vi "sub get keyword value.vi"(8 "error in":errorcluster, 10 "keyword":string[](array[string]), 11 "string":string) -> (0 "error out":errorcluster, 2 "matched pairs (exist)":cluster{"keyword":string, "value":string}[](array[cluster]), 3 "matched pairs (all)":cluster{"keyword":string, "value":string}[](array[cluster]), 5 "remain string":string)   [LabVIEW 2018, in "Data Parser.lvclass"]
uses:
  Data Parser.lvclass
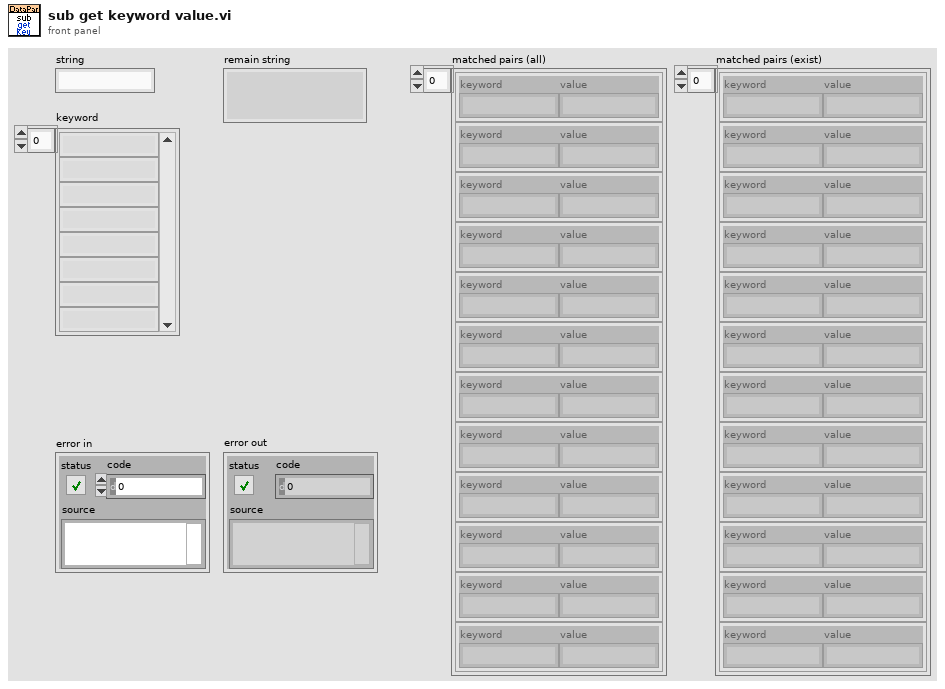
[diagram p1: front panel]
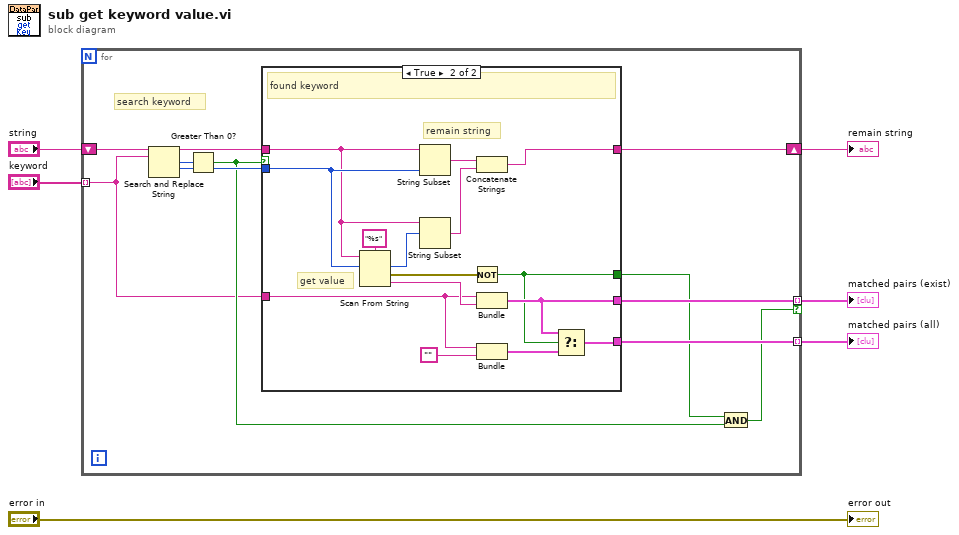
[diagram p0: block diagram]
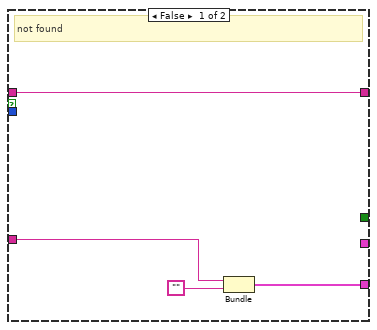
[diagram p2: hidden frame]
diagram:
  n1 = for {
    tunnel: "keyword" -> [w8] mode=indexing
    shift-right: [w14] -> w3
    shift-left: "string" -> [w17]
    tunnel: [w13] -> w6 mode=indexing if=w9
    tunnel: [w12] -> w1 mode=indexing
    # "search keyword"
    n2 = Search and Replace String(input string=w17, search string=w8) -> (result string=w15:string, number of replacements=w11:i32, offset past replacement=w16:i32)  [unwired: 6 in, 1 out]
    n3 = Greater Than 0?(x=w11) -> (x > 0?=w10:bool)
    n4 = case shown="True" w10 {
      tunnel: w16 -> [_ w34]
      tunnel: w15 -> [w21 w33]
      tunnel: [w21 w29] -> w14
      tunnel: [_ w28] -> w13
      tunnel: w8 -> [w19 w27]
      tunnel: [w18 w24] -> w12
      tunnel: [_ w22] -> w7
      frame False {
        # "not found"
        n5 = Bundle("String"=w19, "") -> (w18:cluster{"String":string, string})  [unwired: 1 in]
      }
      frame True {
        # "remain string"
        # "get value"
        # "found keyword"
        n6 = Scan From String(format string="%s", input string=w33, initial scan location=w34) -> (offset past scan=w32:u32, error out=w23:errorcluster, output 1=w35:string)  [unwired: 2 in, 1 out]
        n7 = String Subset(string=w33, length (rest)=w34) -> (substring=w31:string)  [unwired: 1 in]
        n8 = String Subset(string=w33, offset (0)=w32) -> (substring=w30:string)  [unwired: 1 in]
        n9 = Not(x=w23) -> (.not. x?=w22:bool)
        n10 = Concatenate Strings(w31, w30) -> (w29:string)
        n11 = Bundle("String"=w27, w35) -> (w28:cluster{"String":string, string})  [unwired: 1 in]
        n12 = Bundle("String"=w27, "") -> (w25:cluster{"String":string, string})  [unwired: 1 in]
        n13 = Select(t=w28, s=w22, f=w25) -> (s? t:f=w24:cluster{"String":string, string})
      }
    }
    n14 = And(x=w7, y=w10) -> (x .and. y?=w9:bool)
  }
  "matched pairs (exist)" <- w6
  "remain string" <- w3
  "matched pairs (all)" <- w1
  "error out" <- "error in"
